vi "write_message.vi"(8 "error in (no error)":errorcluster, 9 "timeout in ms (-1)":i32, 10 "element":T1, 11 "WebSocket Connection in":refnum<class "WebSocket Connection.lvclass">) -> (0 "error out":errorcluster, 1 "timed out?":bool, 3 "WebSocket Connection out":refnum<class "WebSocket Connection.lvclass">)   [LabVIEW 2019, in "WebSocket Server Toolkit.lvlib" / "WebSocket Connection.lvclass"]
doc: "<b>Description</b> Writes a message to a WebSocket connection."
uses:
  WebSocket Connection.lvclass
  types/frame_data.ctl
  WebSocket Connection.lvclass/WebSocket Connection.ctl
  WebSocket Server Toolkit.lvlib
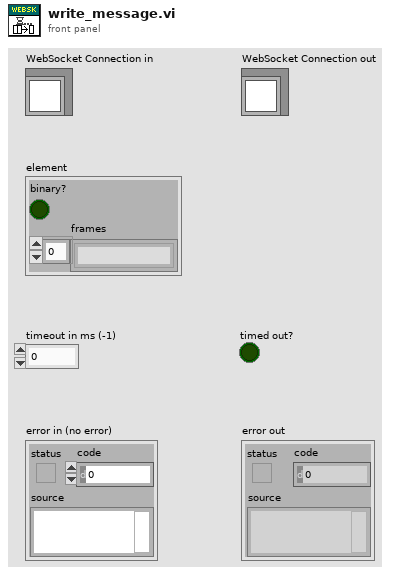
[diagram p1: front panel]
types:
  T1 = typedef "WebSocket Server Toolkit.lvlib/frame_data.ctl" = cluster{"binary?":bool, "frames":string[]}
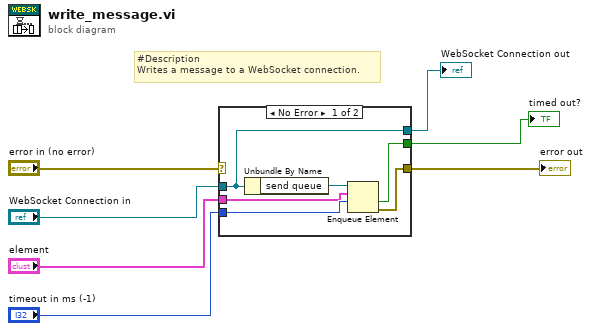
[diagram p0: block diagram]
diagram:
  # "#Description\nWrites a message to a WebSocket connection."
  n1 = case shown="No Error" "error in (no error)" {
    selector: "error in (no error)" -> [_ w15]
    tunnel: [w10 w15] -> w6
    tunnel: [w13 w14] -> w4
    tunnel: "WebSocket Connection in" -> [w13 w14]
    tunnel: "timeout in ms (-1)" -> [w11 _]
    tunnel: [w9 _] -> w2
    tunnel: "element" -> [w8 _]
    frame No Error {
      n2 = Unbundle By Name(w13) -> ("send queue"=w12:refnum<queue>)
      n3 = Enqueue Element(queue=w12, element=w8, timeout in ms (-1)=w11) -> (timed out?=w9:bool, error out=w10:errorcluster)  [unwired: 1 in, 1 out]
    }
    frame Error {
    }
  }
  "error out" <- w6
  "WebSocket Connection out" <- w4
  "timed out?" <- w2
